vi "Post-Build Action - Remove Linux home Dir.vi"(5 "Files Generated by Build":path[](array[path]), 6 "Top Level/Always Included VIs":path[](array[path]), 7 "Destination Path":path, 8 "error in (no error)":errorcluster, 9 "Target Name":string, 10 "Build Specification Name":string, 11 "Project Path":path) -> (0 "error out":errorcluster)   [LabVIEW 2016]
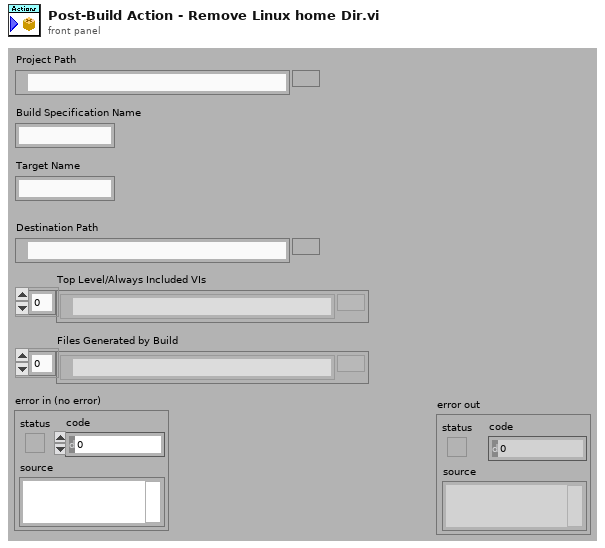
[diagram p1: front panel]
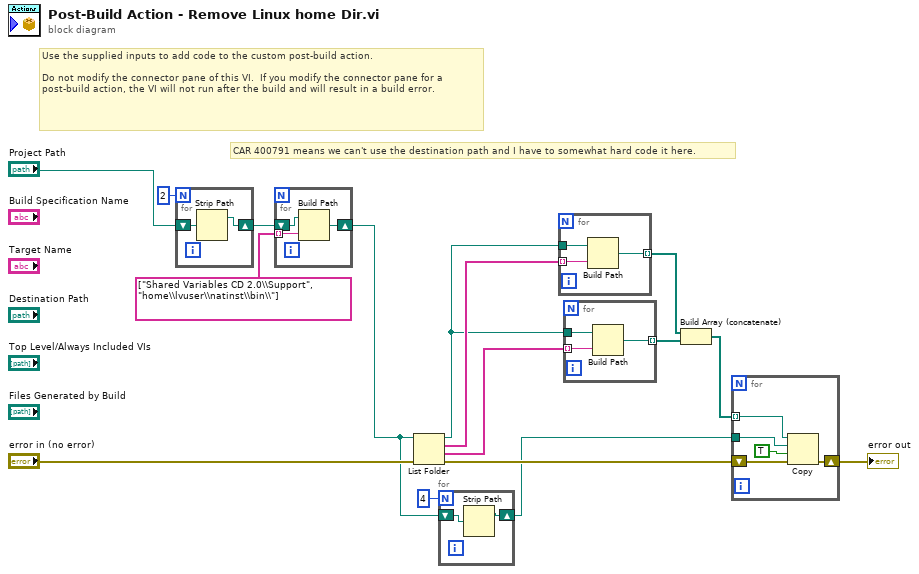
[diagram p0: block diagram]
diagram:
  # "CAR 400791 means we can't use the destination path and I have to somewhat hard code it here."
  # "Use the supplied inputs to add code to the custom post-build action.\n\nDo not modify the connector pane of this VI.  If you modify the connector pane for a post-build action, the VI will not run after the build and will result in a build error."
  n1 = for {
    N: 2 -> [_]
    shift-right: [w17] -> w4
    shift-left: "Project Path" -> [w18]
    n2 = Strip Path(path=w18) -> (stripped path=w17:path)  [unwired: 1 out]
  }
  n3 = for {
    shift-right: [w21] -> w2
    shift-left: w4 -> [w20]
    tunnel: string[] ["Shared Variables CD 2.0\\Support", "home\\lvuser\\natinst\\bin\\"] -> [w19] mode=indexing
    n4 = Build Path(base path=w20, name or relative path=w19) -> (appended path=w21:path)
  }
  n5 = List Folder(path=w2, error in="error in (no error)") -> (path out=w12:path, filenames=w16:string[], folder names=w13:string[], error out=w10:errorcluster)  [unwired: 2 in]
  n6 = for {
    N: 4 -> [_]
    shift-right: [w23] -> w8
    shift-left: w2 -> [w22]
    n7 = Strip Path(path=w22) -> (stripped path=w23:path)  [unwired: 1 out]
  }
  n8 = for {
    tunnel: w16 -> [w25] mode=indexing
    tunnel: w12 -> [w26]
    tunnel: [w24] -> w15 mode=indexing
    n9 = Build Path(base path=w26, name or relative path=w25) -> (appended path=w24:path)
  }
  n10 = for {
    tunnel: w13 -> [w28] mode=indexing
    tunnel: w12 -> [w29]
    tunnel: [w27] -> w11 mode=indexing
    n11 = Build Path(base path=w29, name or relative path=w28) -> (appended path=w27:path)
  }
  n12 = Build Array (concatenate)(w15, w11) -> (w14:path[])
  n13 = for {
    tunnel: w14 -> [w31] mode=indexing
    shift-right: [w32] -> w7
    shift-left: w10 -> [w33]
    tunnel: w8 -> [w30]
    n14 = Copy(8:w33, 9:TRUE ("overwrite (F)"), 10:w30, 11:w31) -> (0:w32:errorcluster)  [unwired: 1 in, 2 out]
  }
  "error out" <- w7
